vi "Configure Measurement Resolution.vi"(8 "error in (no error)":errorcluster {"code" format="%.0x"}, 10 "Measurement Resolution (0: 20 ms)":i32(ring) items=["20 ms", "40 ms"], 11 "VISA resource name":refnum<visa-resource-name>) -> (0 "error out":errorcluster {"code" format="%.0x"}, 3 "VISA resource name out":refnum<visa-resource-name>)   [LabVIEW 2010, in "Agilent N6700 Series.lvlib"]
doc: "Configures the resolution used in setting the time interval between digitized measurements for time intervals above 20.48 microseconds.\n\n<b>Note:</b>\n\nThis VI is used only with models N676xA, N678xA SMU, or models that have Option 054 (High Speed Test Extensions)."
uses:
  Agilent N6700 Series.lvlib
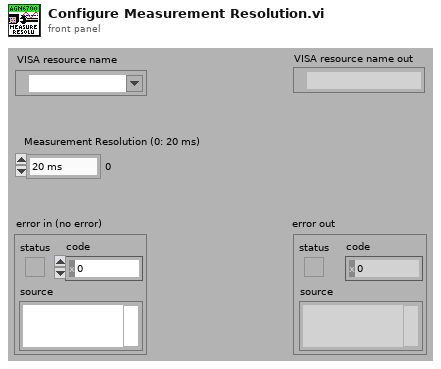
[diagram p1: front panel]
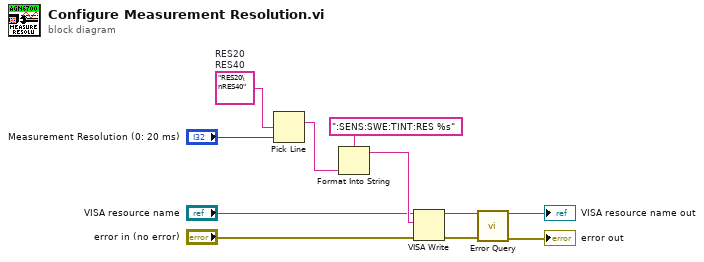
[diagram p0: block diagram]
diagram:
  w11 = "RES20\nRES40"  # RES20 RES40
  n1 = Pick Line(multi-line string=w11, line index="Measurement Resolution (0: 20 ms)") -> (output string=w5:string)  [unwired: 1 in]
  n2 = Format Into String(format string=":SENS:SWE:TINT:RES %s", w5) -> (resulting string=w10:string)  [unwired: 2 in, 1 out]
  n3 = VISA Write(VISA resource name="VISA resource name", write buffer=w10, error in (no error)="error in (no error)") -> (VISA resource name out=w2:refnum<visa-resource-name>, error out=w1:errorcluster)  [unwired: 1 out]
  n4 = call "Error Query.vi"("VISA resource name"=w2, "error in (no error)"=w1) -> ("VISA resource name out"=→"VISA resource name out":refnum<visa-resource-name>, "error out"=→"error out":errorcluster)  [unwired: 10 in, 2 out]
